vi "Destroy Events.vi"(8 "error in (no error)":errorcluster, 11 "Lissajous Viewer in":refnum<class "Lissajous Viewer.lvclass">) -> (0 "error out":errorcluster, 3 "Lissajous Viewer out":refnum<class "Lissajous Viewer.lvclass">)   [LabVIEW 2020, in "Lissajous Viewer.lvlib" / "Lissajous Viewer.lvclass"]
uses:
  Lissajous Viewer.lvclass
  Lissajous Viewer.lvclass/Lissajous Viewer.ctl
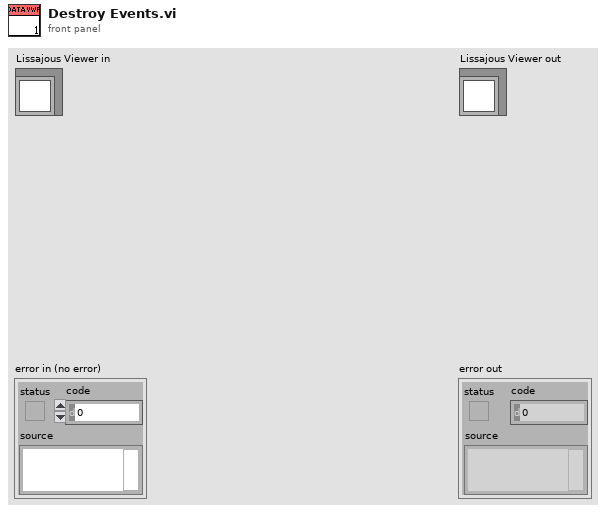
[diagram p1: front panel]
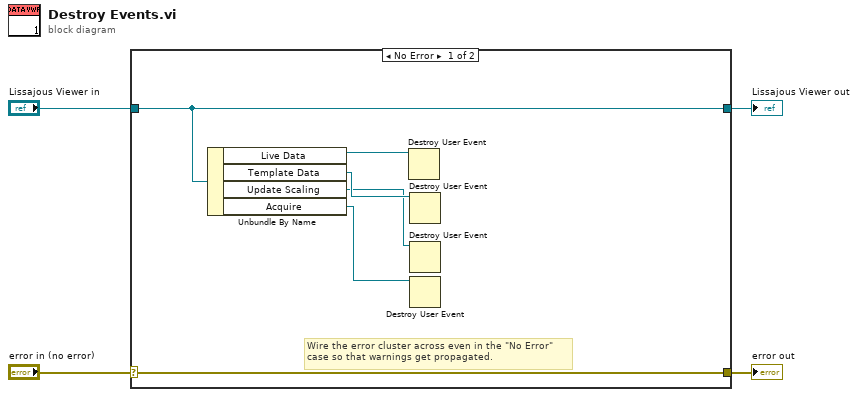
[diagram p0: block diagram]
diagram:
  n1 = case shown="No Error" "error in (no error)" {
    selector: "error in (no error)" -> [w10 w12]
    tunnel: [w10 w12] -> w3
    tunnel: [w9 w11] -> w1
    tunnel: "Lissajous Viewer in" -> [w9 w11]
    frame No Error {
      # "Wire the error cluster across even in the \"No Error\"\ncase so that warnings get propagated."
      n2 = Unbundle By Name(w9) -> ("Live Data"=w8:refnum<user-event>, "Template Data"=w7:refnum<user-event>, "Update Scaling"=w6:refnum<user-event>, "Acquire"=w5:refnum<user-event>)
      n3 = Destroy User Event(user event=w8) -> ()  [unwired: 1 in, 1 out]
      n4 = Destroy User Event(user event=w7) -> ()  [unwired: 1 in, 1 out]
      n5 = Destroy User Event(user event=w6) -> ()  [unwired: 1 in, 1 out]
      n6 = Destroy User Event(user event=w5) -> ()  [unwired: 1 in, 1 out]
    }
    frame Error {
    }
  }
  "error out" <- w3
  "Lissajous Viewer out" <- w1
